vi "StateMachine.vi"() -> ()   [LabVIEW 2019]
uses:
  StatatesEnum.ctl
panel:
  in  "Proc3":bool
  in  "Proc2":bool
  in  "Proc1":bool
  in  "stop":bool
  in  "States":T1=enum."Tineout"
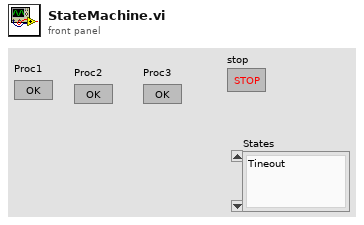
[diagram p1: front panel]
types:
  T1 = typedef "StatatesEnum.ctl" = enum16{"", "Tineout", "Proc1", "Proc2", "Proc3", "Stop"}
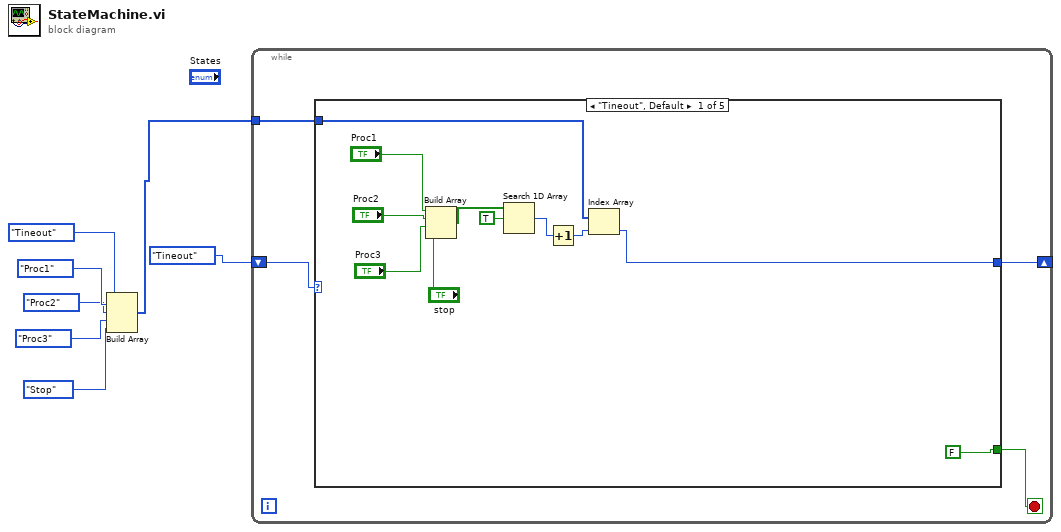
[diagram p0: block diagram]
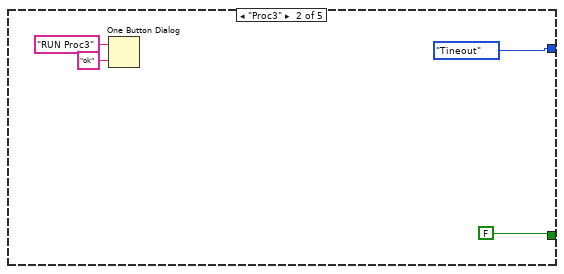
[diagram p2: hidden frame]
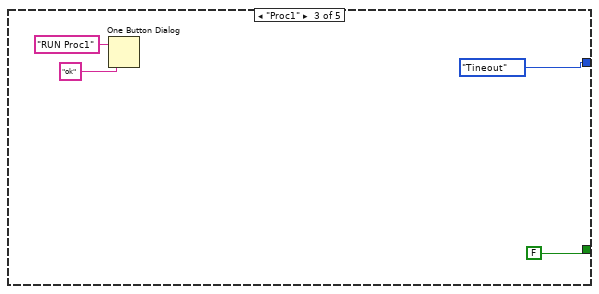
[diagram p3: hidden frame]
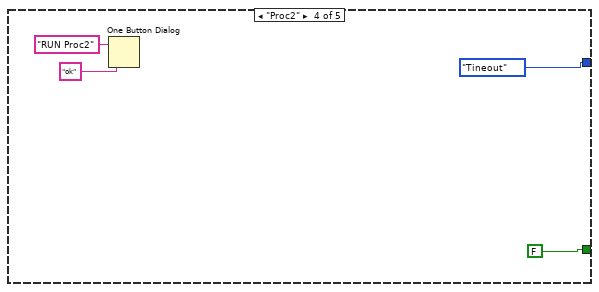
[diagram p4: hidden frame]
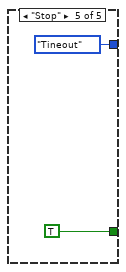
[diagram p5: hidden frame]
diagram:
  n1 = Build Array(StatatesEnum."Tineout" ("States"), StatatesEnum."Proc1" ("States"), StatatesEnum."Proc2" ("States"), StatatesEnum."Proc3" ("States"), StatatesEnum."Stop" ("States")) -> (w3:T1[])
  n2 = while {
    shift-right: [w9] -> _
    shift-left: StatatesEnum."Tineout" ("States") -> [w11]
    tunnel: w3 -> [w10]
    stop <- w8 stop-if-true
    n3 = case shown="\"Tineout\", Default" w11 {
      tunnel: w10 -> [w16 _ _ _ _]
      tunnel: [w15 StatatesEnum."Tineout" ("States") StatatesEnum."Tineout" ("States") StatatesEnum."Tineout" ("States") StatatesEnum."Tineout" ("States")] -> w9
      tunnel: [FALSE FALSE FALSE FALSE TRUE] -> w8
      frame "Tineout", Default {
        n4 = Build Array("Proc1", "Proc2", "Proc3", "stop") -> (w20:bool[])
        n5 = Search 1D Array(1D array=w20, element=TRUE) -> (index of element=w18:i32)  [unwired: 1 in]
        n6 = Increment(x=w18) -> (x+1=w17:i32)
        n7 = Index Array(array=w16, index=w17) -> (element=w15:T1)
      }
      frame "Proc3" {
        n8 = One Button Dialog(message="RUN Proc3", button name ("OK")="ok") -> ()  [unwired: 1 out]
      }
      frame "Proc1" {
        n9 = One Button Dialog(message="RUN Proc1", button name ("OK")="ok") -> ()  [unwired: 1 out]
      }
      frame "Proc2" {
        n10 = One Button Dialog(message="RUN Proc2", button name ("OK")="ok") -> ()  [unwired: 1 out]
      }
      frame "Stop" {
      }
    }
  }
